vi "test-profiled-PID-input-output.vi"(8 "error in (no error)":errorcluster) -> (0 "error out":errorcluster, 3 "All Tests Passed":bool)   [LabVIEW 2019]
uses:
  <vilib>/Rock Robotics/WPI/ThirdParty/JAS_Junk/TrajLib/ProfiledPIDController_NewPeriod.vi
  <vilib>/Rock Robotics/WPI/ThirdParty/JAS_Junk/TrajLib/PIDController_SetPID.vi
  <vilib>/Rock Robotics/WPI/ThirdParty/JAS_Junk/TrajLib/ProfiledPIDController_SetGoal_PosOnly.vi
  <vilib>/Rock Robotics/WPI/ThirdParty/JAS_Junk/TrajLib/ProfiledPIDController_Calculate_Meas.vi
  <vilib>/Rock Robotics/WPI/ThirdParty/JAS_Junk/TrajLib/PIDController_GetPeriod.vi
  <vilib>/Rock Robotics/WPI/ThirdParty/JAS_Junk/TrajLib/PIDController_EnableContinousInput.vi
  <vilib>/Rock Robotics/WPI/ThirdParty/JAS_Junk/TrajLib/TrapProfState_New.vi
  <vilib>/Rock Robotics/WPI/ThirdParty/JAS_Junk/TrajLib/ProfiledPIDController_Reset.vi
  <vilib>/Rock Robotics/WPI/ThirdParty/JAS_Junk/TrajLib/PIDController_NewPeriod.vi
  <vilib>/Rock Robotics/SystemInterfaces/NetworkCommunication/NetComm_UsageReport_report.vi
  <vilib>/Rock Robotics/WPI/ThirdParty/JAS_Junk/TrajLib/ProfiledPIDController_SetGoal.vi
  <vilib>/Rock Robotics/WPI/ThirdParty/JAS_Junk/TrajLib/PIDController_Calculate_SP_PV.vi
  <vilib>/Rock Robotics/WPI/ThirdParty/JAS_Junk/TrajLib/TrapProfile_New.vi
  <vilib>/Rock Robotics/WPI/ThirdParty/JAS_Junk/TrajLib/TrapProfile_Calculate.vi
  <vilib>/Rock Robotics/WPI/ThirdParty/JAS_Junk/TrajLib/ControllerUtil_GetModulusError.vi
  <vilib>/Rock Robotics/WPI/ThirdParty/JAS_Junk/TrajLib/PIDController_Reset.vi
  <vilib>/Rock Robotics/WPI/ThirdParty/JAS_Junk/TrajLib/PIDController_SetSetpoint.vi
  <vilib>/Rock Robotics/WPI/ThirdParty/JAS_Junk/TrajLib/PIDController_Calculate_PV.vi
  <vilib>/Rock Robotics/WPI/ThirdParty/JAS_Junk/TrajLib/TrapProfile_ShouldFlipAcceleration.vi
  <vilib>/Rock Robotics/WPI/ThirdParty/JAS_Junk/TrajLib/TrapProfile_Direct.vi
  <vilib>/Rock Robotics/WPI/ThirdParty/JAS_Junk/TrajLib/Util_LibraryGlobals.vi
  <vilib>/Rock Robotics/WPI/ThirdParty/JAS_Junk/TrajLib/Trajectory_Library.lvlib
panel:
  out "Test Passed 6":bool
  out "Test Passed 5":bool
  out "Test Passed 4":bool
  out "Test Passed 3":bool
  out "Test Passed 2":bool
  out "Test Passed 1":bool
  out "Test Passed 0":bool
  # "Profiled PID  Input  / Ouptut"
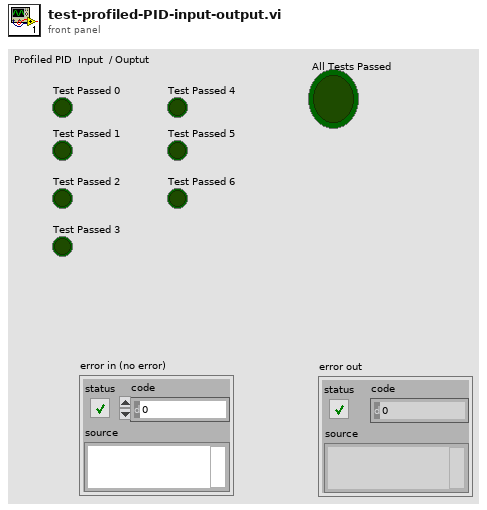
[diagram p1: front panel]
types:
  T1 = typedef "Trajectory_Library.lvlib/TRAPEZOID_PROFILE_CONSTRAINT.ctl" = cluster{"MaxVelocity":dbl, "MaxAcceleration":dbl}
  T2 = typedef "Trajectory_Library.lvlib/PROFILED_PID_CONTROLLER.ctl" = cluster{"Controller":T3, "Goal":T4, "Setpoint":T4, "Constraint":T1}
  T3 = typedef "Trajectory_Library.lvlib/PID_CONTROLLER.ctl" = cluster{"Kp":dbl, "Ki":dbl, "Kd":dbl, "Period":dbl, "Max_Integral":dbl, "Min_Integral":dbl, "Max_Input":dbl, "Min_Input":dbl, "Continuous":bool, "PositionError":dbl, "VelocityError":dbl, "PrevError":dbl, "TotalError":dbl, "PositionTolerance":dbl, "VelocityTolerance":dbl, "SetPoint":dbl, "Kf":dbl, "Prev_Deriv":dbl, "Prev_Deriv 2":dbl, "DerivativeFilter":bool, "Min_Output":dbl, "Max_Output":dbl, "Prev_F_P":dbl, "Prev_F_P_2":dbl, "AntiWindupActive":bool, "Measurement":dbl}
  T4 = typedef "Trajectory_Library.lvlib/TRAPEZOID_PROFILE_STATE.ctl" = cluster{"Position":dbl, "Velocity":dbl}
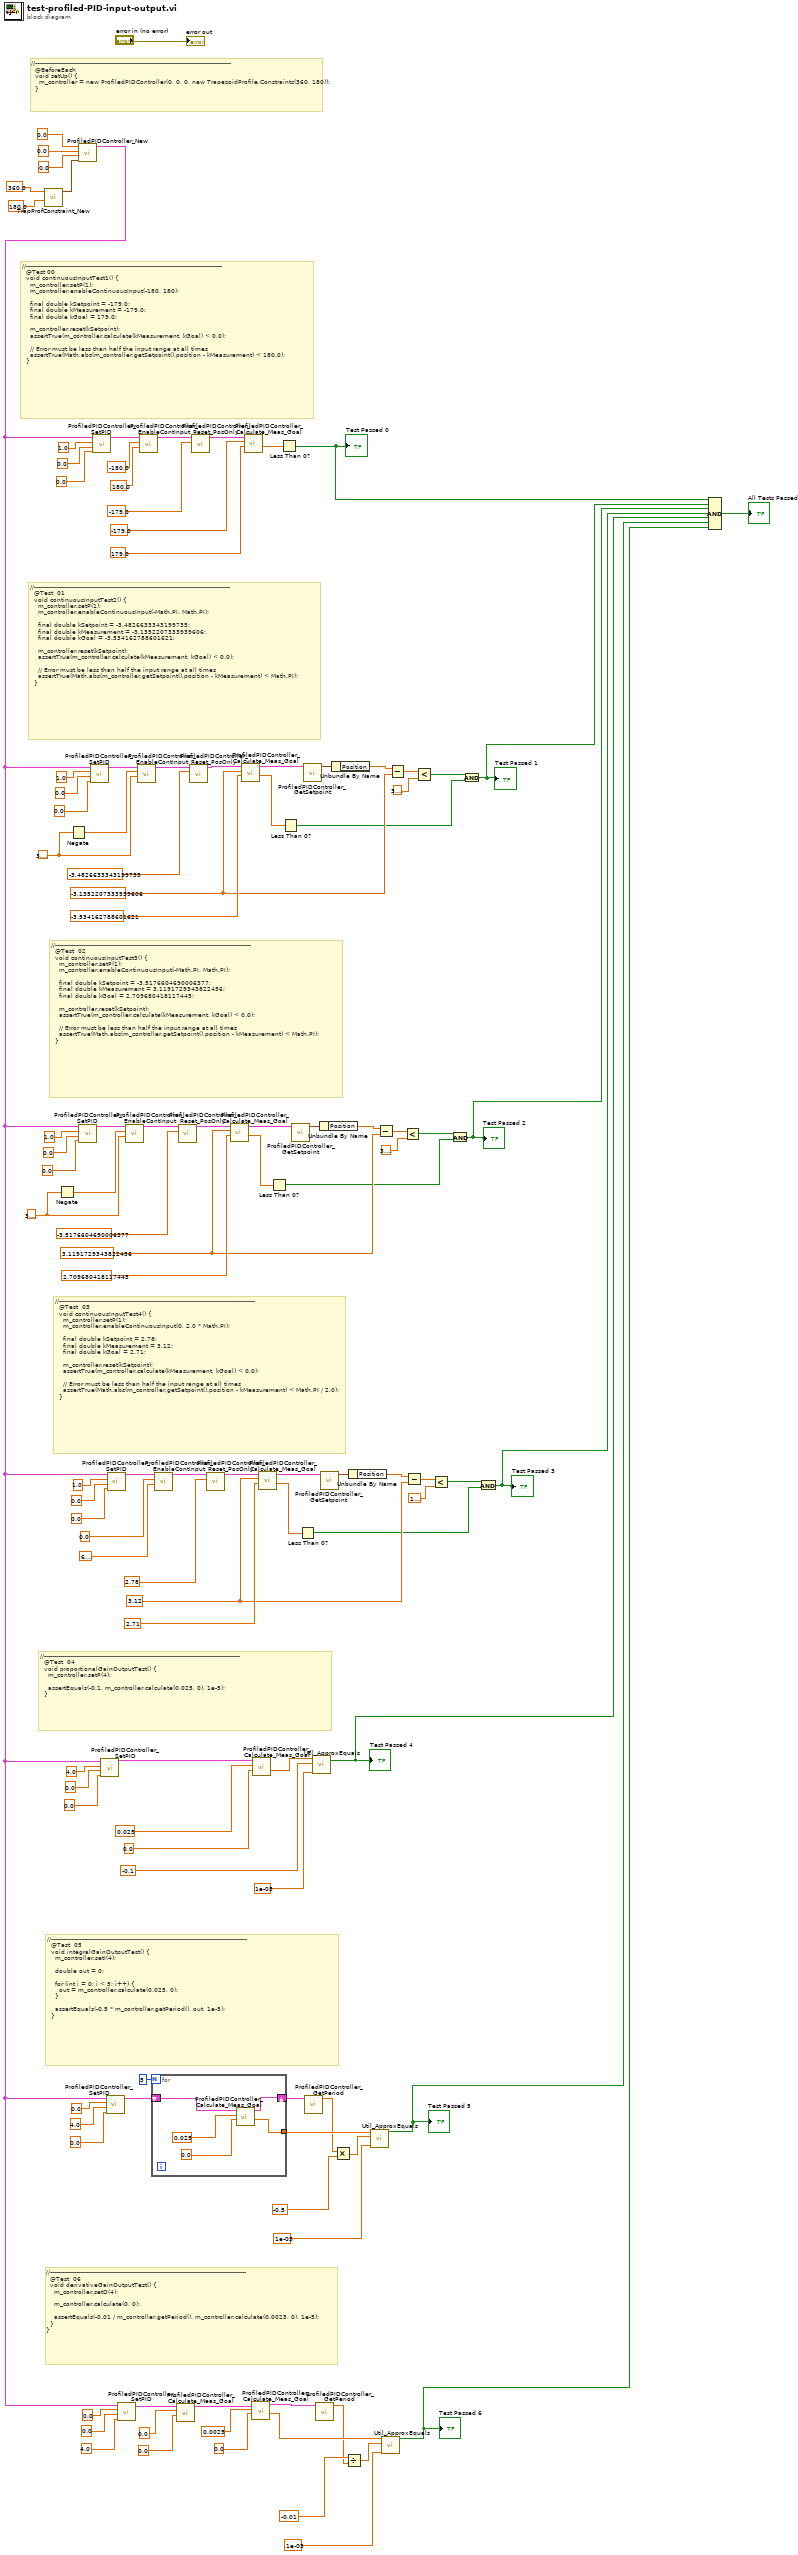
[diagram p0: block diagram]
diagram:
  w51 = 3.12 ("PV-Measurement")
  w72 = 3.141592653589793
  w68 = 3.1191729343822456 ("PV-Measurement")
  w91 = 3.141592653589793
  w87 = -3.1352207333939606 ("PV-Measurement")
  # "//--------------------------------------------------------------------------------------------------\n  @Test  05\n  void integralGainOutputTest() {\n    m_controller.setI(4);\n\n    double out = 0;\n\n    for (int i = 0; i < 5; i++) {\n      out = m_controller.calculate(0.025, 0);\n    }\n\n    assertEquals(-0.5 * m_controller.getPeriod(), out, 1e-5);\n  }"
  # "//--------------------------------------------------------------------------------------------------\n  @Test  04\n  void proportionalGainOutputTest() {\n    m_controller.setP(4);\n\n    assertEquals(-0.1, m_controller.calculate(0.025, 0), 1e-5);\n  }"
  # "//--------------------------------------------------------------------------------------------------\n  @Test  03\n  void continuousInputTest4() {\n    m_controller.setP(1);\n    m_controller.enableContinuousInput(0, 2.0 * Math.PI);\n\n    final double kSetpoint = 2.78;\n    final double kMeasurement = 3.12;\n    final double kGoal = 2.71;\n\n    m_controller.reset(kSetpoint);\n    assertTrue(m_controller.calculate(kMeasurement, kGoal) < 0.0);\n\n    // Error must be less than half the input range at all times\n    assertTrue(Math.abs(m_controller.getSetpoint().position - kMeasurement) < Math.PI / 2.0);\n  }"
  # "//--------------------------------------------------------------------------------------------------\n  @Test  02\n  void continuousInputTest3() {\n    m_controller.setP(1);\n    m_controller.enableContinuousInput(-Math.PI, Math.PI);\n\n    final double kSetpoint = -3.5176604690006377;\n    final double kMeasurement = 3.1191729343822456;\n    final double kGoal = 2.709680418117445;\n\n    m_controller.reset(kSetpoint);\n    assertTrue(m_controller.calculate(kMeasurement, kGoal) < 0.0);\n\n    // Error must be less than half the input range at all times\n    assertTrue(Math.abs(m_controller.getSetpoint().position - kMeasurement) < Math.PI);\n  }"
  # "//--------------------------------------------------------------------------------------------------\n  @Test  01\n  void continuousInputTest2() {\n    m_controller.setP(1);\n    m_controller.enableContinuousInput(-Math.PI, Math.PI);\n\n    final double kSetpoint = -3.4826633343199735;\n    final double kMeasurement = -3.1352207333939606;\n    final double kGoal = -3.534162788601621;\n\n    m_controller.reset(kSetpoint);\n    assertTrue(m_controller.calculate(kMeasurement, kGoal) < 0.0);\n\n    // Error must be less than half the input range at all times\n    assertTrue(Math.abs(m_controller.getSetpoint().position - kMeasurement) < Math.PI);\n  }"
  # "//--------------------------------------------------------------------------------------------------\n  @Test 00\n  void continuousInputTest1() {\n    m_controller.setP(1);\n    m_controller.enableContinuousInput(-180, 180);\n\n    final double kSetpoint = -179.0;\n    final double kMeasurement = -179.0;\n    final double kGoal = 179.0;\n\n    m_controller.reset(kSetpoint);\n    assertTrue(m_controller.calculate(kMeasurement, kGoal) < 0.0);\n\n    // Error must be less than half the input range at all times\n    assertTrue(Math.abs(m_controller.getSetpoint().position - kMeasurement) < 180.0);\n  }"
  # "//--------------------------------------------------------------------------------------------------\n  @BeforeEach\n  void setUp() {\n    m_controller = new ProfiledPIDController(0, 0, 0, new TrapezoidProfile.Constraints(360, 180));\n  }"
  # "//--------------------------------------------------------------------------------------------------\n  @Test  06\n  void derivativeGainOutputTest() {\n    m_controller.setD(4);\n\n    m_controller.calculate(0, 0);\n\n    assertEquals(-0.01 / m_controller.getPeriod(), m_controller.calculate(0.0025, 0), 1e-5);\n  }\n}"
  n1 = call <vilib>:"TrapProfConstraint_New.vi"("Max Accel"=180.0, "Max Speed (M/S)"=360.0 ("Max Accel")) -> ("TRAPEZOID_PROFILE_CONSTRAINT"=w115:T1)  [unwired: 9 in]
  n2 = Negate(x=w72) -> (-x=w73:dbl)
  n3 = Negate(x=w91) -> (-x=w92:dbl)
  n4 = call <vilib>:"ProfiledPIDController_New.vi"("Constraints"=w115, "Kd"=0.0 ("Kp"), "Ki"=0.0 ("Kp"), "Kp"=0.0) -> ("PROFILED_PID_CONTROLLER"=w17:T2)  [unwired: 7 in]
  n5 = call <vilib>:"ProfiledPIDController_SetPID.vi"("Kd"=0.0, "Ki"=0.0, "Kp"=1.0, "in PROFILED_PID_CONTROLLER"=w17) -> ("out PROFILED_PID_CONTROLLER"=w80:T2)  [unwired: 7 in]
  n6 = call <vilib>:"ProfiledPIDController_SetPID.vi"("Kd"=0.0, "Ki"=0.0, "Kp"=1.0, "in PROFILED_PID_CONTROLLER"=w17) -> ("out PROFILED_PID_CONTROLLER"=w99:T2)  [unwired: 7 in]
  n7 = call <vilib>:"ProfiledPIDController_SetPID.vi"("Kd"=0.0, "Ki"=0.0, "Kp"=1.0, "in PROFILED_PID_CONTROLLER"=w17) -> ("out PROFILED_PID_CONTROLLER"=w110:T2)  [unwired: 7 in]
  n8 = call <vilib>:"ProfiledPIDController_SetPID.vi"("Kd"=0.0, "Ki"=0.0, "Kp"=4.0, "in PROFILED_PID_CONTROLLER"=w17) -> ("out PROFILED_PID_CONTROLLER"=w40:T2)  [unwired: 7 in]
  n9 = call <vilib>:"ProfiledPIDController_SetPID.vi"("Kd"=0.0, "Ki"=4.0, "Kp"=0.0, "in PROFILED_PID_CONTROLLER"=w17) -> ("out PROFILED_PID_CONTROLLER"=w32:T2)  [unwired: 7 in]
  n10 = call <vilib>:"ProfiledPIDController_SetPID.vi"("Kd"=0.0, "Ki"=0.0, "Kp"=1.0, "in PROFILED_PID_CONTROLLER"=w17) -> ("out PROFILED_PID_CONTROLLER"=w61:T2)  [unwired: 7 in]
  n11 = call <vilib>:"ProfiledPIDController_SetPID.vi"("Kd"=4.0, "Ki"=0.0, "Kp"=0.0, "in PROFILED_PID_CONTROLLER"=w17) -> ("out PROFILED_PID_CONTROLLER"=w12:T2)  [unwired: 7 in]
  n12 = call <vilib>:"ProfiledPIDController_EnableContInput.vi"("MaxInput"=w72, "MinInput"=w73, "in PROFILED_PID_CONTROLLER"=w80) -> ("out PROFILED_PID_CONTROLLER"=w79:T2)  [unwired: 8 in]
  n13 = call <vilib>:"ProfiledPIDController_EnableContInput.vi"("MaxInput"=w91, "MinInput"=w92, "in PROFILED_PID_CONTROLLER"=w99) -> ("out PROFILED_PID_CONTROLLER"=w98:T2)  [unwired: 8 in]
  n14 = call <vilib>:"ProfiledPIDController_EnableContInput.vi"("MaxInput"=180.0, "MinInput"=-180.0, "in PROFILED_PID_CONTROLLER"=w110) -> ("out PROFILED_PID_CONTROLLER"=w107:T2)  [unwired: 8 in]
  n15 = for {
    N: 5 -> [_]
    tunnel: [w122] -> w31
    shift-right: [w121] -> w28
    shift-left: w32 -> [w124]
    n16 = call <vilib>:"ProfiledPIDController_Calculate_Meas_Goal.vi"("SP-Goal"=0.0, "PV-Measurement"=0.025 ("Position"), "in PROFILED_PID_CONTROLLER"=w124) -> ("CO-ControlOutput"=w122:dbl, "out PROFILED_PID_CONTROLLER"=w121:T2)  [unwired: 7 in]
  }
  n17 = call <vilib>:"ProfiledPIDController_EnableContInput.vi"("MaxInput"=6.283185307179586, "MinInput"=0.0, "in PROFILED_PID_CONTROLLER"=w61) -> ("out PROFILED_PID_CONTROLLER"=w60:T2)  [unwired: 8 in]
  n18 = call <vilib>:"ProfiledPIDController_Calculate_Meas_Goal.vi"("SP-Goal"=0.0, "PV-Measurement"=0.0 ("Position"), "in PROFILED_PID_CONTROLLER"=w12) -> ("out PROFILED_PID_CONTROLLER"=w11:T2)  [unwired: 7 in, 1 out]
  n19 = call <vilib>:"ProfiledPIDController_Reset_PosOnly.vi"("Position"=-3.5176604690006377, "in PROFILED_PID_CONTROLLER"=w79) -> ("out PROFILED_PID_CONTROLLER"=w77:T2)  [unwired: 9 in]
  n20 = call <vilib>:"ProfiledPIDController_Reset_PosOnly.vi"("Position"=-3.4826633343199735, "in PROFILED_PID_CONTROLLER"=w98) -> ("out PROFILED_PID_CONTROLLER"=w96:T2)  [unwired: 9 in]
  n21 = call <vilib>:"ProfiledPIDController_Reset_PosOnly.vi"("Position"=-179.0, "in PROFILED_PID_CONTROLLER"=w107) -> ("out PROFILED_PID_CONTROLLER"=w105:T2)  [unwired: 9 in]
  n22 = call <vilib>:"ProfiledPIDController_Reset_PosOnly.vi"("Position"=2.78, "in PROFILED_PID_CONTROLLER"=w60) -> ("out PROFILED_PID_CONTROLLER"=w58:T2)  [unwired: 9 in]
  n23 = call <vilib>:"ProfiledPIDController_Calculate_Meas_Goal.vi"("SP-Goal"=2.709680418117445, "PV-Measurement"=w68, "in PROFILED_PID_CONTROLLER"=w77) -> ("CO-ControlOutput"=w75:dbl, "out PROFILED_PID_CONTROLLER"=w71:T2)  [unwired: 7 in]
  n24 = call <vilib>:"ProfiledPIDController_Calculate_Meas_Goal.vi"("SP-Goal"=-3.534162788601621, "PV-Measurement"=w87, "in PROFILED_PID_CONTROLLER"=w96) -> ("CO-ControlOutput"=w94:dbl, "out PROFILED_PID_CONTROLLER"=w90:T2)  [unwired: 7 in]
  n25 = call <vilib>:"ProfiledPIDController_Calculate_Meas_Goal.vi"("SP-Goal"=179.0, "PV-Measurement"=-179.0, "in PROFILED_PID_CONTROLLER"=w105) -> ("CO-ControlOutput"=w102:dbl)  [unwired: 7 in, 1 out]
  n26 = call <vilib>:"ProfiledPIDController_Calculate_Meas_Goal.vi"("SP-Goal"=0.0, "PV-Measurement"=0.0025 ("Position"), "in PROFILED_PID_CONTROLLER"=w11) -> ("CO-ControlOutput"=w21:dbl, "out PROFILED_PID_CONTROLLER"=w19:T2)  [unwired: 7 in]
  n27 = call <vilib>:"ProfiledPIDController_Calculate_Meas_Goal.vi"("SP-Goal"=0.0, "PV-Measurement"=0.025 ("Position"), "in PROFILED_PID_CONTROLLER"=w40) -> ("CO-ControlOutput"=w38:dbl)  [unwired: 7 in, 1 out]
  n28 = call <vilib>:"ProfiledPIDController_Calculate_Meas_Goal.vi"("SP-Goal"=2.71, "PV-Measurement"=w51, "in PROFILED_PID_CONTROLLER"=w58) -> ("CO-ControlOutput"=w56:dbl, "out PROFILED_PID_CONTROLLER"=w54:T2)  [unwired: 7 in]
  n29 = Less Than 0?(x=w75) -> (x < 0?=w64:bool)
  n30 = Less Than 0?(x=w102) -> (x < 0?=w8:bool)
  "Test Passed 0" <- w8
  n31 = Less Than 0?(x=w94) -> (x < 0?=w83:bool)
  n32 = call <vilib>:"ProfiledPIDController_GetSetpoint.vi"("in PROFILED_PID_CONTROLLER"=w71) -> ("Setpoint"=w70:T4)  [unwired: 10 in]
  n33 = Less Than 0?(x=w56) -> (x < 0?=w47:bool)
  n34 = call <vilib>:"ProfiledPIDController_GetSetpoint.vi"("in PROFILED_PID_CONTROLLER"=w90) -> ("Setpoint"=w89:T4)  [unwired: 10 in]
  n35 = call <vilib>:"ProfiledPIDController_GetPeriod.vi"("in PROFILED_PID_CONTROLLER"=w28) -> ("Period"=w26:dbl)  [unwired: 10 in]
  n36 = call <vilib>:"Util_ApproxEquals.vi"("Tolerance"=1e-05, "Value 2"=-0.1 ("PV-Measurement"), "Value 1"=w38) -> ("ApproxEquals"=w4:bool)  [unwired: 8 in]
  "Test Passed 4" <- w4
  n37 = call <vilib>:"ProfiledPIDController_GetPeriod.vi"("in PROFILED_PID_CONTROLLER"=w19) -> ("Period"=w9:dbl)  [unwired: 10 in]
  n38 = Unbundle By Name(w70) -> ("Position"=w69:dbl)
  n39 = call <vilib>:"ProfiledPIDController_GetSetpoint.vi"("in PROFILED_PID_CONTROLLER"=w54) -> ("Setpoint"=w53:T4)  [unwired: 10 in]
  n40 = Unbundle By Name(w89) -> ("Position"=w88:dbl)
  n41 = Multiply(x=w26, y=-0.5 ("PV-Measurement")) -> (x*y=w27:dbl)
  n42 = Divide(x=-0.01 ("PV-Measurement"), y=w9) -> (x/y=w18:dbl)
  n43 = Unbundle By Name(w53) -> ("Position"=w52:dbl)
  n44 = call <vilib>:"Util_ApproxEquals.vi"("Tolerance"=1e-05, "Value 2"=w27, "Value 1"=w31) -> ("ApproxEquals"=w3:bool)  [unwired: 8 in]
  "Test Passed 5" <- w3
  n45 = Subtract(x=w69, y=w68) -> (x-y=w67:dbl)
  n46 = call <vilib>:"Util_ApproxEquals.vi"("Tolerance"=1e-05, "Value 2"=w18, "Value 1"=w21) -> ("ApproxEquals"=w2:bool)  [unwired: 8 in]
  "Test Passed 6" <- w2
  n47 = Subtract(x=w88, y=w87) -> (x-y=w86:dbl)
  n48 = Less?(x=w67, y=3.141592653589793) -> (x < y?=w65:bool)
  n49 = Subtract(x=w52, y=w51) -> (x-y=w50:dbl)
  n50 = Less?(x=w86, y=3.141592653589793) -> (x < y?=w84:bool)
  n51 = Less?(x=w50, y=1.5707963267948966) -> (x < y?=w48:bool)
  n52 = And(x=w65, y=w64) -> (x .and. y?=w6:bool)
  "Test Passed 2" <- w6
  n53 = And(x=w84, y=w83) -> (x .and. y?=w7:bool)
  "Test Passed 1" <- w7
  n54 = And(x=w48, y=w47) -> (x .and. y?=w5:bool)
  "Test Passed 3" <- w5
  n55 = Compound Arithmetic op=AND(w8, w7, w6, w5, w4, w3, w2) -> (→"All Tests Passed":bool)
  "error out" <- "error in (no error)"
